vi "TCP Discoverable Server Test.vi"() -> ()   [LabVIEW 2020]
panel:
  in  "stop":bool
  out "Discover":bool
  out "IP Address":string="169.254.245.221"
  in  "Port":i32=4900
  out "Error":bool
  out "Command":string
  out "Connected":bool
  out "Ready":bool
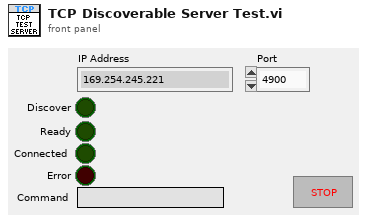
[diagram p1: front panel]
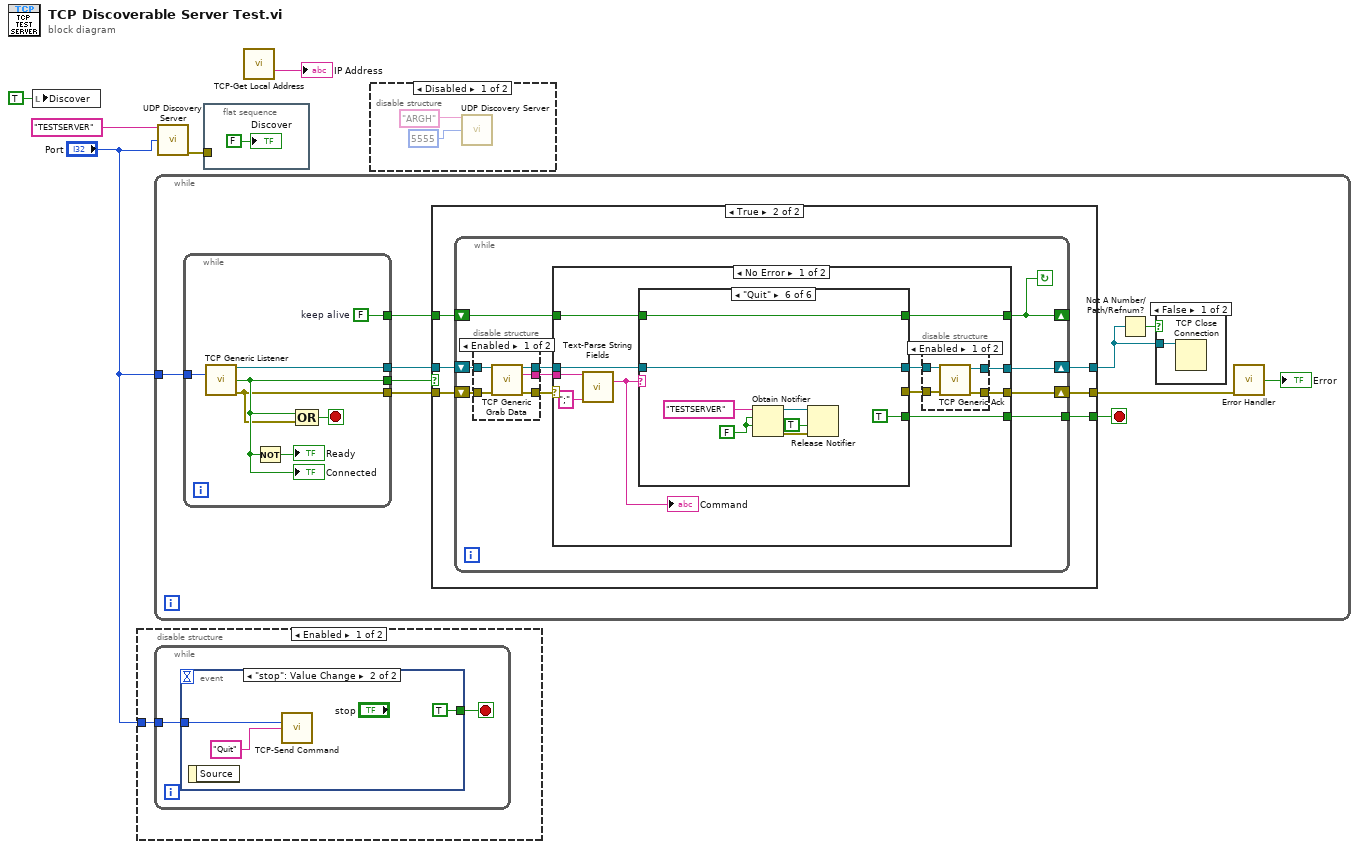
[diagram p0: block diagram]
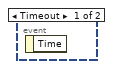
[diagram p3: hidden frame]
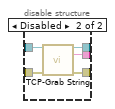
[diagram p6: hidden frame]
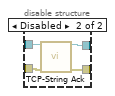
[diagram p7: hidden frame]
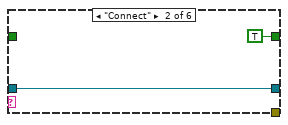
[diagram p9: hidden frame]
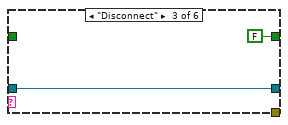
[diagram p10: hidden frame]
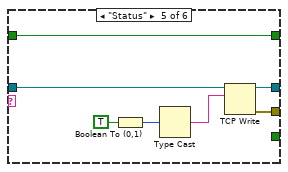
[diagram p12: hidden frame]
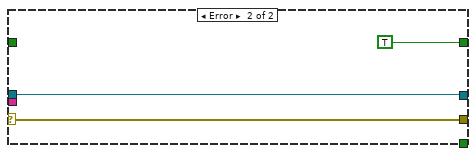
[diagram p13: hidden frame]
diagram:
  n1 = local write "Discover"(TRUE ("Discover")) -> ()
  n2 = disable-structure shown="Enabled" {
    disable-tunnel: "Port" -> [w6 _]
    frame Enabled {
      n3 = while {
        tunnel: w6 -> [w7]
        stop <- w8 stop-if-true
        n4 = event shown="[1] \"stop\": Value Change" {
          selector: _ -> [_ _]
          dyn-events: _ -> [_ _]
          timeout: _ -> [_ _]
          tunnel: [_ TRUE ("stop")] -> w8
          tunnel: w7 -> [_ w10]
          event Timeout {
            n5 = event-data() -> ()  [unwired: 1 in, 1 out]
          }
          event "stop": Value Change {
            n6 = event-data() -> ()  [unwired: 1 in, 1 out]
            n7 = call "TCP-Send Command.vi"("Port"=w10, "Command"="Quit") -> ()  [unwired: 13 in, 1 out]
          }
        }
      }
    }
    frame Disabled {
    }
  }
  n8 = while {
    tunnel: "Port" -> [w21]
    stop <- w16 stop-if-true
    n9 = while {
      tunnel: w21 -> [w101]
      tunnel: [w97] -> w20
      tunnel: [w100] -> w19
      tunnel: [w96] -> w13
      tunnel: [w95] -> w12
      stop <- w99 stop-if-true
      w95 = FALSE  # keep alive
      n10 = call "TCP Generic Listener.vi"("port"=w101) -> ("connection ID"=w100:refnum<k5>, "Connected?"=w97:bool, "error out"=w96:errorcluster)  [unwired: 12 in]
      "Connected" <- w97
      n11 = Not(x=w97) -> (.not. x?=→"Ready":bool)
      n12 = Compound Arithmetic op=OR(w97, w96) -> (w99:bool)
    }
    n13 = case shown="True" w20 {
      tunnel: w13 -> [w22 w28]
      tunnel: w19 -> [w23 w29]
      tunnel: [w23 w27] -> w17
      tunnel: [w22 w26] -> w14
      tunnel: [_ w25] -> w16
      tunnel: w12 -> [_ w24]
      frame False {
      }
      frame True {
        n14 = while {
          tunnel: [w34] -> w25
          shift-right: [w31] -> w27
          shift-left: w29 -> [w39]
          shift-right: [w30] -> w26
          shift-left: w28 -> [w38]
          shift-right: [w32] -> _
          shift-left: w24 -> [w33]
          stop <- w32 continue-if-true
          n15 = disable-structure shown="Enabled" {
            disable-tunnel: w39 -> [w44 w49]
            disable-tunnel: w38 -> [w43 w48]
            disable-tunnel: [w42 w46] -> w37
            disable-tunnel: [w41 w45] -> w36
            disable-tunnel: [w40 w47] -> w35
            frame Enabled {
              n16 = call "TCP Generic Grab Data.vi"("connection ID"=w44, "error in (no error)"=w43) -> ("connection ID out"=w40:refnum<k5>, "data out"=w42:string, "error out"=w41:errorcluster)  [unwired: 11 in]
            }
            frame Disabled {
              n17 = call "TCP-Grab String.vi"("connection ID"=w49, "error in (no error)"=w48) -> ("connection ID out"=w47:refnum<k5>, "data out"=w46:string, "error out"=w45:errorcluster)  [unwired: 11 in]
            }
          }
          n18 = case shown="No Error" w36 {
            selector: w36 -> [_ w94]
            tunnel: w37 -> [w60 _]
            tunnel: w35 -> [w59 w92]
            tunnel: [w50 w94] -> w30
            tunnel: [w58 _] -> w34
            tunnel: w33 -> [w55 _]
            tunnel: [w54 TRUE] -> w32
            tunnel: [w51 w92] -> w31
            frame No Error {
              n19 = call "Text-Parse String Fields.vi"("String"=w60, "Separator"=";") -> ("element"=w56:string)  [unwired: 8 in, 5 out]
              "Command" <- w56
              n20 = case shown="\"Quit\"" w56 {
                tunnel: w59 -> [w70 w72 w74 w76 w81 w91]
                tunnel: [w70 w72 w74 w76 w83 w91] -> w53
                tunnel: [_ _ _ _ w82 _] -> w52
                tunnel: [_ _ _ _ _ TRUE] -> w58
                tunnel: w55 -> [w69 _ _ w75 w77 w89]
                tunnel: [w69 TRUE FALSE w75 w77 w89] -> w54
                frame "", Default {
                }
                frame "Connect" {
                }
                frame "Disconnect" {
                }
                frame "Ping" {
                }
                frame "Status" {
                  n21 = Boolean To (0,1)(Boolean=TRUE) -> (0, 1=w79:i16)
                  n22 = Type Cast(x=w79) -> (*(type *) &x=w80:string)  [unwired: 1 in]
                  n23 = TCP Write(connection ID=w81, data in=w80) -> (connection ID out=w83:refnum<k5>, error out=w82:errorcluster)  [unwired: 2 in, 1 out]
                }
                frame "Quit" {
                  w85 = FALSE
                  n24 = Obtain Notifier(name (unnamed)="TESTSERVER", notification data type=w85, create if not found? (T)=w85) -> (notifier out=w87:refnum<notifier>, error out=w86:errorcluster)  [unwired: 1 in, 1 out]
                  n25 = Release Notifier(notifier=w87, force destroy? (F)=TRUE, error in (no error)=w86) -> ()  [unwired: 3 out]
                }
              }
              n26 = disable-structure shown="Enabled" {
                disable-tunnel: w53 -> [w64 w68]
                disable-tunnel: w52 -> [w63 w65]
                disable-tunnel: [w62 w67] -> w51
                disable-tunnel: [w61 w66] -> w50
                frame Enabled {
                  n27 = call "TCP Generic Ack.vi"("error in (no error)"=w63, "connection ID"=w64) -> ("error out"=w61:errorcluster, "connection ID out"=w62:refnum<k5>)  [unwired: 8 in]
                }
                frame Disabled {
                  n28 = call "TCP-String Ack.vi"("connection ID"=w68, "error in (no error)"=w65) -> ("connection ID out"=w67:refnum<k5>, "error out"=w66:errorcluster)  [unwired: 12 in]
                }
              }
            }
            frame Error {
            }
          }
        }
      }
    }
    n29 = Not A Number/Path/Refnum?(number/path/refnum=w17) -> (NaN/Path/Refnum?=w18:bool)
    n30 = case shown="False" w18 {
      tunnel: w17 -> [w102 _]
      frame False {
        n31 = TCP Close Connection(connection ID=w102) -> ()  [unwired: 2 in, 2 out]
      }
      frame True {
      }
    }
    n32 = call "Error Handler.vi"("error in (no error)"=w14) -> ("error?"=→"Error":bool)  [unwired: 12 in, 2 out]
  }
  n33 = call "UDP Discovery Server.vi"("Name"="TESTSERVER", "Port"="Port") -> ("error out"=w4:errorcluster)  [unwired: 13 in]
  n34 = flat-sequence {
    tunnel: w4 -> [_]
    frame #0 {
      "Discover" <- FALSE ("Discover")
    }
  }
  n35 = call "TCP-Get Local Address.vi"() -> ("address"=→"IP Address":string)  [unwired: 14 in, 1 out]
  n36 = disable-structure shown="Disabled" {
    frame Disabled {
      n37 = call "UDP Discovery Server.vi"("Name"="ARGH", "Port"=u16 5555) -> ()  [unwired: 13 in, 1 out]
    }
    frame Enabled {
    }
  }
